vi "Configure Library in Memory for Build.vi"(7 "target name (My Computer)":string="My Computer", 9 "enable debugging? (F)":bool, 10 "save VIs? (T)":bool=TRUE, 11 "library name":string="DSF Core.lvlib") -> (0 "error out":errorcluster)   [LabVIEW 2017, in "Build Automation.lvlib"]
uses:
  Build Automation.lvlib
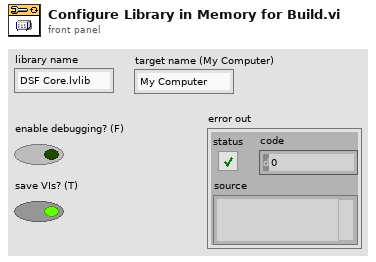
[diagram p1: front panel]
types:
  T1 = enum16{"Share clones between instances", "Preallocate clone for each instance"}
  T2 = cluster{"Status Message":refnum<data-value>, "Progress":refnum<data-value>, "Stop":refnum<data-value>}
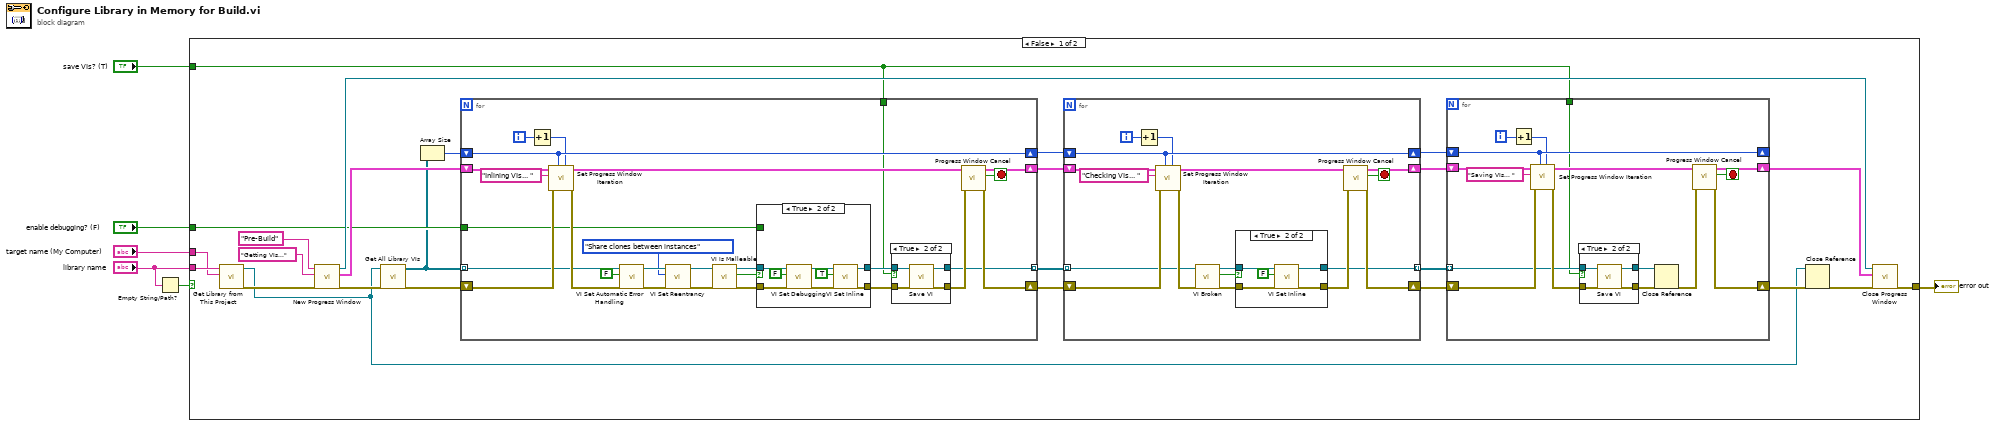
[diagram p0: block diagram]
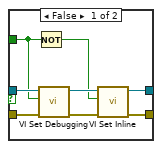
[diagram p3: hidden frame]
diagram:
  n1 = Empty String/Path?(string/path="library name") -> (empty?=w3:bool)
  n2 = case shown="False" w3 {
    tunnel: [w28 _] -> w6
    tunnel: "enable debugging? (F)" -> [w27 _]
    tunnel: "library name" -> [w10 _]
    tunnel: "save VIs? (T)" -> [w8 _]
    tunnel: "target name (My Computer)" -> [w9 _]
    frame False {
      n3 = call "Get Library from This Project.vi"("Target Name (My Computer)"=w9, "Library Name"=w10) -> ("error out"=w12:errorcluster, "Library Refnum"=w11:refnum<vi>)  [unwired: 8 in]
      n4 = call "New Progress Window.vi"("error in (no error)"=w12, "Initial Message"="Getting VIs...", "Window Title"="Pre-Build" ("WindowTitle")) -> ("error out"=w30:errorcluster, "DVRs"=w29:T2, "VI refnum"=w31:refnum<vi>)  [unwired: 6 in]
      n5 = call "Get All Library VIs.vi"("error in (no error)"=w30, "library ref"=w11) -> ("error out"=w32:errorcluster, "vi refs"=w25:refnum<vi>[])  [unwired: 8 in]
      n6 = Array Size(array=w25) -> (size(s)=w26:i32)
      n7 = for {
        tunnel: w25 -> [w42] mode=indexing
        shift-right: [w57] -> w23
        shift-left: w29 -> [w47]
        shift-right: [w43] -> w21
        shift-left: w32 -> [w45]
        tunnel: w27 -> [w41]
        tunnel: [w33] -> w22 mode=indexing
        shift-right: [w40] -> w24
        shift-left: w26 -> [w40]
        tunnel: w8 -> [w34]
        i -> [w59]
        stop <- w58 stop-if-true
        n8 = Increment(x=w59) -> (x+1=w39:i32)
        n9 = call "Set Progress Window Iteration.vi"("current iteration"=w39, "total iterations"=w40, "error in (no error)"=w45, "Status Message"="Inlining VIs... ", "DVRs in"=w47) -> ("error out"=w44:errorcluster, "DVRs out"=w46:T2)  [unwired: 5 in]
        n10 = call "VI Set Automatic Error Handling.vi"("error in (no error)"=w44, "Automatic Error Handling"=FALSE, "vi ref in"=w42) -> ("error out"=w54:errorcluster, "vi ref out"=w55:refnum<vi>)  [unwired: 7 in]
        n11 = call "VI Set Reentrancy.vi"("error in (no error)"=w54, "Reentrancy Type"=T1."Share clones between instances", "vi ref in"=w55) -> ("error out"=w51:errorcluster, "vi ref out"=w52:refnum<vi>)  [unwired: 7 in]
        n12 = call "VI Is Malleable.vi"("error in (no error)"=w51, "vi ref in"=w52) -> ("error out"=w50:errorcluster, "malleable VI?"=w48:bool, "vi ref out"=w49:refnum<vi>)  [unwired: 7 in]
        n13 = case shown="True" w48 {
          tunnel: [w71 w79] -> w36
          tunnel: [w70 w78] -> w37
          tunnel: w50 -> [w67 w76]
          tunnel: w49 -> [w68 w77]
          tunnel: w41 -> [w66 _]
          frame False {
            n14 = Not(x=w66) -> (.not. x?=w69:bool)
            n15 = call "VI Set Debugging.vi"("error in (no error)"=w67, "Allow Debugging"=w66, "vi ref in"=w68) -> ("error out"=w72:errorcluster, "vi ref out"=w73:refnum<vi>)  [unwired: 7 in]
            n16 = call "VI Set Inline.vi"("error in (no error)"=w72, "Inline VI"=w69, "vi ref in"=w73) -> ("error out"=w70:errorcluster, "vi ref out"=w71:refnum<vi>)  [unwired: 7 in]
          }
          frame True {
            n17 = call "VI Set Debugging.vi"("error in (no error)"=w76, "Allow Debugging"=FALSE, "vi ref in"=w77) -> ("error out"=w80:errorcluster, "vi ref out"=w81:refnum<vi>)  [unwired: 7 in]
            n18 = call "VI Set Inline.vi"("error in (no error)"=w80, "Inline VI"=TRUE, "vi ref in"=w81) -> ("error out"=w78:errorcluster, "vi ref out"=w79:refnum<vi>)  [unwired: 7 in]
          }
        }
        n19 = case shown="True" w34 {
          tunnel: w37 -> [w60 w65]
          tunnel: [w61 w64] -> w33
          tunnel: [w60 w63] -> w35
          tunnel: w36 -> [w61 w62]
          frame False {
          }
          frame True {
            n20 = call "Save VI.vi"("error in (no error)"=w65, "vi ref in"=w62) -> ("error out"=w63:errorcluster, "vi ref out"=w64:refnum<vi>)  [unwired: 8 in]
          }
        }
        n21 = call "Progress Window Cancel.vi"("error in (no error)"=w35, "DVRs in"=w46) -> ("error out"=w43:errorcluster, "cancelled"=w58:bool, "DVRs out"=w57:T2)  [unwired: 7 in]
      }
      n22 = for {
        tunnel: w22 -> [w87] mode=indexing
        shift-right: [w96] -> w20
        shift-left: w23 -> [w95]
        shift-right: [w92] -> w18
        shift-left: w21 -> [w93]
        shift-right: [w91] -> w19
        shift-left: w24 -> [w91]
        tunnel: [w82] -> w17 mode=indexing
        i -> [w98]
        stop <- w97 stop-if-true
        n23 = Increment(x=w98) -> (x+1=w90:i32)
        n24 = call "Set Progress Window Iteration.vi"("current iteration"=w90, "total iterations"=w91, "error in (no error)"=w93, "Status Message"="Checking VIs... ", "DVRs in"=w95) -> ("error out"=w88:errorcluster, "DVRs out"=w94:T2)  [unwired: 5 in]
        n25 = call "VI Broken.vi"("error in (no error)"=w88, "vi ref in"=w87) -> ("error out"=w85:errorcluster, "broken?"=w84:bool, "vi ref out"=w86:refnum<vi>)  [unwired: 7 in]
        n26 = case shown="True" w84 {
          tunnel: [w100 w105] -> w82
          tunnel: [w99 w104] -> w83
          tunnel: w85 -> [w99 w103]
          tunnel: w86 -> [w100 w101]
          frame False {
          }
          frame True {
            n27 = call "VI Set Inline.vi"("error in (no error)"=w103, "Inline VI"=FALSE, "vi ref in"=w101) -> ("error out"=w104:errorcluster, "vi ref out"=w105:refnum<vi>)  [unwired: 7 in]
          }
        }
        n28 = call "Progress Window Cancel.vi"("error in (no error)"=w83, "DVRs in"=w94) -> ("error out"=w92:errorcluster, "cancelled"=w97:bool, "DVRs out"=w96:T2)  [unwired: 7 in]
      }
      n29 = for {
        tunnel: w17 -> [w107] mode=indexing
        shift-right: [w119] -> w16
        shift-left: w20 -> [w118]
        shift-right: [w115] -> w14
        shift-left: w18 -> [w116]
        shift-right: [w114] -> _
        shift-left: w19 -> [w114]
        tunnel: w8 -> [w106]
        i -> [w121]
        stop <- w120 stop-if-true
        n30 = Increment(x=w121) -> (x+1=w113:i32)
        n31 = call "Set Progress Window Iteration.vi"("current iteration"=w113, "total iterations"=w114, "error in (no error)"=w116, "Status Message"="Saving VIs... ", "DVRs in"=w118) -> ("error out"=w108:errorcluster, "DVRs out"=w117:T2)  [unwired: 5 in]
        n32 = case shown="True" w106 {
          tunnel: w108 -> [w122 w127]
          tunnel: [w123 w126] -> w111
          tunnel: [w122 w125] -> w110
          tunnel: w107 -> [w123 w124]
          frame False {
          }
          frame True {
            n33 = call "Save VI.vi"("error in (no error)"=w127, "vi ref in"=w124) -> ("error out"=w125:errorcluster, "vi ref out"=w126:refnum<vi>)  [unwired: 8 in]
          }
        }
        n34 = Close Reference(reference=w111, error in (no error)=w110) -> (error out=w109:errorcluster)
        n35 = call "Progress Window Cancel.vi"("error in (no error)"=w109, "DVRs in"=w117) -> ("error out"=w115:errorcluster, "cancelled"=w120:bool, "DVRs out"=w119:T2)  [unwired: 7 in]
      }
      n36 = Close Reference(reference=w11, error in (no error)=w14) -> (error out=w13:errorcluster)
      n37 = call "Close Progress Window.vi"("error in (no error)"=w13, "DVRs in"=w16, "VI refnum"=w31) -> ("error out"=w28:errorcluster)  [unwired: 8 in]
    }
    frame True {
    }
  }
  "error out" <- w6
